vi "Init Arrays.vi"(8 "error in (no error)":errorcluster, 11 "Graph Manager in":refnum<class "Graph Manager.lvclass">) -> (0 "error out":errorcluster, 3 "Graph Manager out":refnum<class "Graph Manager.lvclass">)   [LabVIEW 2016, in "Graph Manager.lvclass"]
uses:
  Graph Manager.lvclass
  Graph Manager.lvclass/Graph Manager.ctl
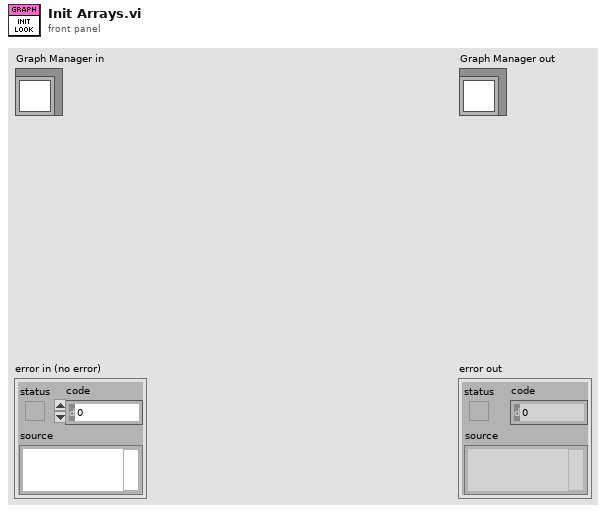
[diagram p1: front panel]
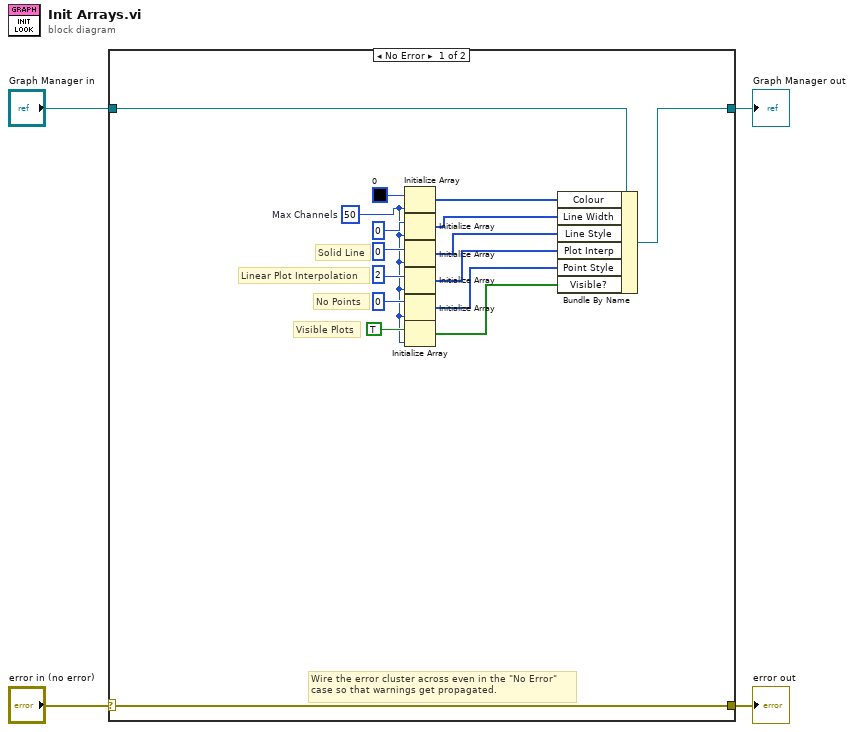
[diagram p0: block diagram]
diagram:
  n1 = case shown="No Error" "error in (no error)" {
    selector: "error in (no error)" -> [w20 w22]
    tunnel: [w20 w22] -> w3
    tunnel: [w14 w21] -> w1
    tunnel: "Graph Manager in" -> [w15 w21]
    frame No Error {
      w5 = 50  # Max Channels
      # "Visible Plots"
      # "No Points"
      # "Solid Line"
      # "Linear Plot Interpolation"
      # "Wire the error cluster across even in the \"No Error\"\ncase so that warnings get propagated."
      n2 = Initialize Array(u32 0, w5) -> (w19:u32[])
      n3 = Initialize Array(u8 0 ("width"), w5) -> (w17:u8[])
      n4 = Initialize Array(u8 0 ("width"), w5) -> (w13:u8[])
      n5 = Initialize Array(u8 2 ("width"), w5) -> (w12:u8[])
      n6 = Initialize Array(u8 0 ("width"), w5) -> (w11:u8[])
      n7 = Initialize Array(TRUE, w5) -> (w7:bool[])
      n8 = Bundle By Name(cluster=w15, "Colour"=w19, "Line Width"=w17, "Line Style"=w13, "Plot Interp"=w12, "Point Style"=w11, "Visible?"=w7) -> (w14:refnum<class "Graph Manager.lvclass">)
    }
    frame Error {
    }
  }
  "error out" <- w3
  "Graph Manager out" <- w1
